vi "create_table.vi"() -> ()   [LabVIEW 2020]
uses:
  <vilib>/drjdpowell/SQLite Library/SQL Connection/Open (string).vi
  <vilib>/drjdpowell/SQLite Library/SQL Connection/Execute SQL (1D String).vi
  <vilib>/drjdpowell/SQLite Library/SQL Connection/Connection.lvclass
  <vilib>/drjdpowell/SQLite Library/SQLite.lvlib
panel:
  out "Result Set":string[](array[string])
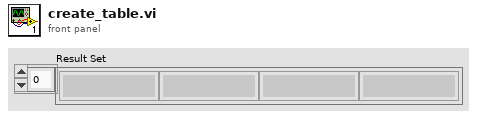
[diagram p1: front panel]
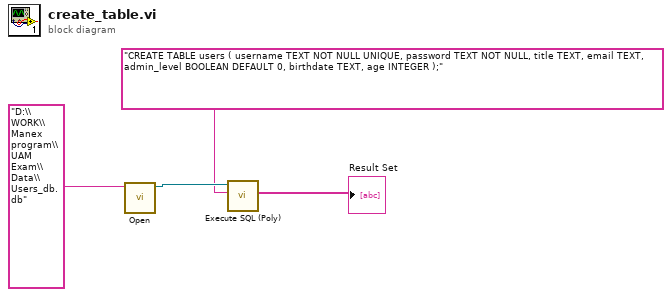
[diagram p0: block diagram]
diagram:
  n1 = call-poly <vilib>:"Open.vi"("db file"="D:\\WORK\\Manex program\\UAM Exam\\Data\\Users_db.db") -> ("SQLite Connection"=w3:refnum<class "Connection.lvclass">)  [unwired: 9 in, 1 out]
  n2 = call-poly <vilib>:"Execute SQL (Poly).vi"("SQL"="CREATE TABLE users ( username TEXT NOT NULL UNIQUE, password TEXT NOT NULL, title TEXT, email TEXT, admin_level BOOLEAN DEFAULT 0, birthdate TEXT, age INTEGER );", "SQLite Connection in"=w3) -> ("Result Set"=→"Result Set":string[])  [unwired: 6 in, 3 out]
